vi "Example Instrument.setMagnet.vi"(8 "error in (no error)":errorcluster, 9 "timeout in ms (1000)":i32 min=0, 10 "setMagnet":dbl, 11 "Example Instrument":refnum<class "Example Instrument.lvclass">) -> (0 "error out":errorcluster, 1 "timed out?":bool, 2 "notification":dbl, 3 "Example Instrument out":refnum<class "Example Instrument.lvclass">)   [LabVIEW 2016, in "Example Instrument.lvclass"]
doc: "---------------------------------------------------------------\nJKI State Machine Objects™\nhttp://jki.net/state-machine-objects/\nCopyright (C) 2005-2015, JKI <info@jki.net>\nALL RIGHTS RESERVEDJKI State Machine Objects (SMO) 1.0.0.4\nJKI - JKI\nCopyright (c) 2015, JKI"
uses:
  Example Instrument.lvclass
  Typedefs/PrivateEvents--Example Instrument.setMagnet.ctl
  Example Instrument.lvclass/Example Instrument.ctl
panel:
  # "For instructions on how to use the JKI State Machine Objects, examples and video tutorials, visit:\nhttp://jki.net/state-machine-objects/\n\nJKI State Machine Objects™\nhttp://jki.net/state-machine-objects/\nCopyright (C) 2005-2015, JKI <info@jki.net>\nALL RIGHTS RESERVED"
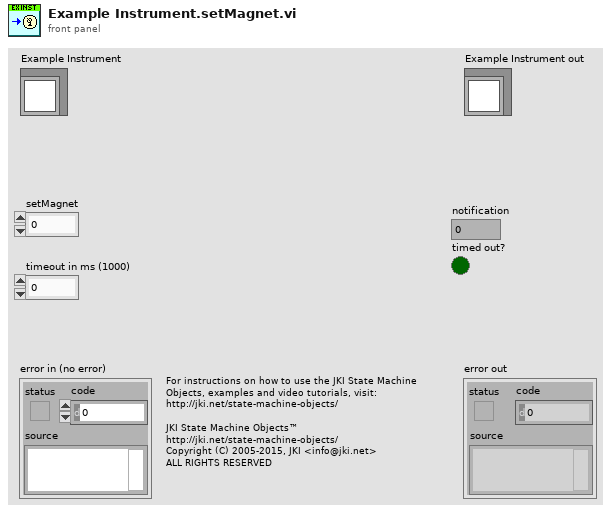
[diagram p1: front panel]
types:
  T1 = typedef "Example Instrument.lvclass/PrivateEvents--Example Instrument.setMagnet.ctl" = cluster{"setMagnet":dbl, "notifier":refnum<notifier>}
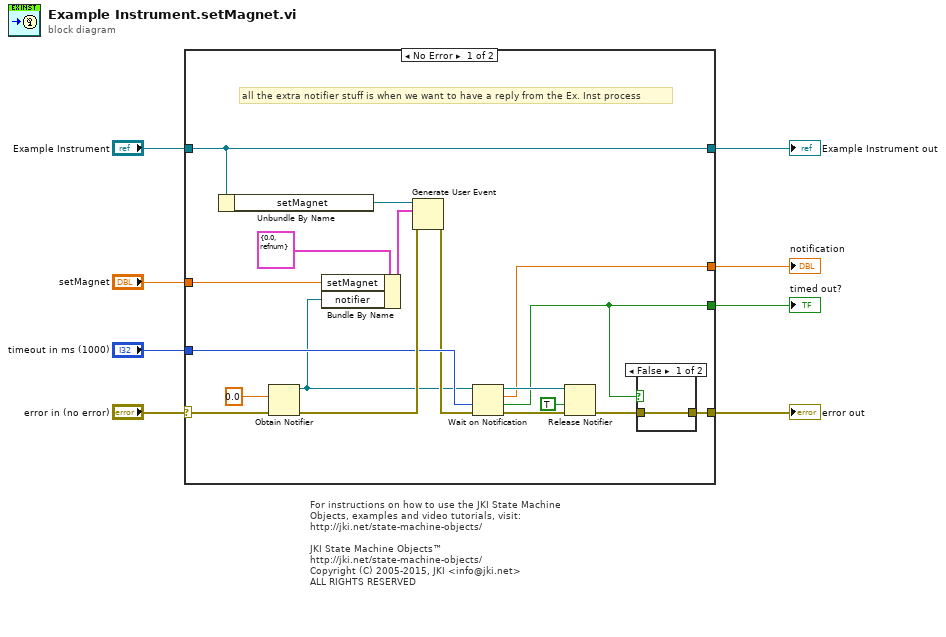
[diagram p0: block diagram]
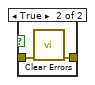
[diagram p2: hidden frame]
diagram:
  # "For instructions on how to use the JKI State Machine Objects, examples and video tutorials, visit:\nhttp://jki.net/state-machine-objects/\n\nJKI State Machine Objects™\nhttp://jki.net/state-machine-objects/\nCopyright (C) 2005-2015, JKI <info@jki.net>\nALL RIGHTS RESERVED"
  n1 = case shown="No Error" "error in (no error)" {
    selector: "error in (no error)" -> [w20 w31]
    tunnel: [w11 w31] -> w7
    tunnel: [w25 w30] -> w8
    tunnel: "Example Instrument" -> [w25 w30]
    tunnel: "setMagnet" -> [w9 _]
    tunnel: "timeout in ms (1000)" -> [w19 _]
    tunnel: [w14 _] -> w2
    tunnel: [w10 _] -> w1
    frame No Error {
      # "all the extra notifier stuff is when we want to have a reply from the Ex. Inst process"
      n2 = Unbundle By Name(w25) -> ("setMagnet"=w26:refnum<user-event>)
      n3 = Obtain Notifier(notification data type=0.0, error in (no error)=w20) -> (notifier out=w15:refnum<notifier>, error out=w21:errorcluster)  [unwired: 2 in, 1 out]
      n4 = Bundle By Name(cluster=T1 {"setMagnet"=0.0, "notifier"=refnum} ("setMagnet"), "setMagnet"=w9, "notifier"=w15) -> (w22:T1)
      n5 = Generate User Event(user event=w26, event data cluster=w22, error in=w21) -> (error out=w18:errorcluster)  [unwired: 1 in, 1 out]
      n6 = Wait on Notification(notifier=w15, timeout in ms (-1)=w19, error in (no error)=w18) -> (notifier out=w17:refnum<notifier>, notification=w14:dbl, timed out?=w10:bool, error out=w16:errorcluster)  [unwired: 1 in]
      n7 = Release Notifier(notifier=w17, force destroy? (F)=TRUE, error in (no error)=w16) -> (error out=w12:errorcluster)  [unwired: 2 out]
      n8 = case shown="False" w10 {
        tunnel: w12 -> [w27 w29]
        tunnel: [w27 w28] -> w11
        frame False {
        }
        frame True {
          n9 = call <vilib>:"Clear Errors.vi"("error in (no error)"=w29) -> ("error out"=w28:errorcluster)  [unwired: 5 in, 1 out]
        }
      }
    }
    frame Error {
    }
  }
  "error out" <- w7
  "Example Instrument out" <- w8
  "notification" <- w2
  "timed out?" <- w1
